vi "HEWH GET General Information.vi"(0 "Stop Custom Draw":bool, 5 "error in (no error)":errorcluster) -> (14 "UI Loop Status":bool, 15 "Stop Draw Status":bool, 16 "Pressurize Tank Status":bool, 17 "Message":string, 19 "error out":errorcluster)   [LabVIEW 2019]
uses:
  Utility/Type Definitions/UTILITY Notifier.ctl
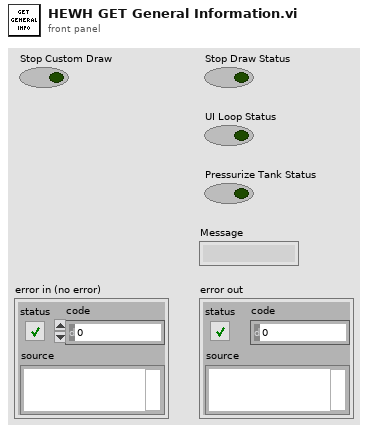
[diagram p1: front panel]
types:
  T1 = typedef "UTILITY Notifier.ctl" = enum16{"Set", "Read", "Release Ref"}
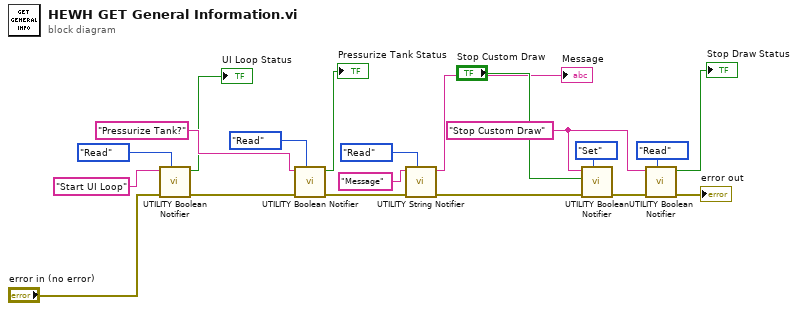
[diagram p0: block diagram]
diagram:
  w16 = "Stop Custom Draw" ("name (unnamed)")
  n1 = call "UTILITY Boolean Notifier.vi"("Status"=UTILITY_Notifier."Read", "error in (no error)"="error in (no error)", "name (unnamed)"="Start UI Loop") -> ("error out"=w8:errorcluster, "latest READ notification"=→"UI Loop Status":bool)  [unwired: 7 in]
  n2 = call "UTILITY Boolean Notifier.vi"("Status"=UTILITY_Notifier."Read", "error in (no error)"=w8, "name (unnamed)"="Pressurize Tank?") -> ("error out"=w14:errorcluster, "latest READ notification"=→"Pressurize Tank Status":bool)  [unwired: 7 in]
  n3 = call "UTILITY String Notifier.vi"("Status"=UTILITY_Notifier."Read", "error in (no error)"=w14, "name (unnamed)"="Message") -> ("error out"=w20:errorcluster, "latest notification"=→"Message":string)  [unwired: 7 in]
  n4 = call "UTILITY Boolean Notifier.vi"("Status"=UTILITY_Notifier."Set", "error in (no error)"=w20, "Set Status"="Stop Custom Draw", "name (unnamed)"=w16) -> ("error out"=w15:errorcluster)  [unwired: 6 in, 1 out]
  n5 = call "UTILITY Boolean Notifier.vi"("Status"=UTILITY_Notifier."Read", "error in (no error)"=w15, "name (unnamed)"=w16) -> ("error out"=→"error out":errorcluster, "latest READ notification"=→"Stop Draw Status":bool)  [unwired: 7 in]
